vi "JYMoveFW.vi"(8 "error in (no error)":errorcluster, 10 "Filter Index":i32(ring)=1 items=["Filter 1"=1, "Empty"=2, "Empty"=3, "Empty"=4, "Filter 2"=5, "Filter 3"=6], 11 "FW RefNum In":refnum<k7>) -> (0 "error out":errorcluster, 3 "FW RefNum Out":refnum<k7>)   [LabVIEW 2009]
doc: "Sets the Filter Wheel position based off of numbered index (1-6).\n\n1- Clear Filter\n2- No Filter\n3- No Filter\n4- No Filter\n5- Orange Filter\n6- Clear Filter"
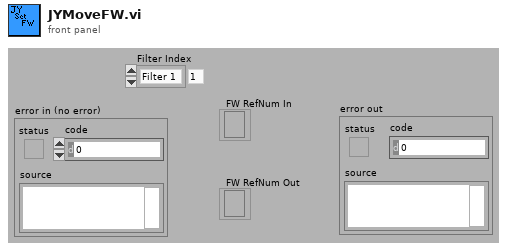
[diagram p1: front panel]
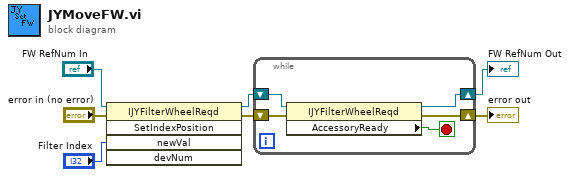
[diagram p0: block diagram]
diagram:
  n1 = invoke class="IJYFilterWheelReqd" method="SetIndexPosition"(reference="FW RefNum In", error in="error in (no error)", "newVal"="Filter Index") -> (reference out=w6:refnum<k7>, error out=w5:errorcluster)  [unwired: 2 in, 3 out]
  n2 = while {
    shift-right: [w10] -> w4
    shift-left: w6 -> [w12]
    shift-right: [w9] -> w3
    shift-left: w5 -> [w11]
    stop <- w8 stop-if-true
    n3 = property class="IJYFilterWheelReqd"(reference=w12, error in=w11) -> (reference out=w10:refnum<k7>, error out=w9:errorcluster, "AccessoryReady"=w8:bool)
  }
  "FW RefNum Out" <- w4
  "error out" <- w3
